vi "Abort Sequence-Ganging.vi"(8 "error in":errorcluster, 11 "Abort Sequence - Ganging":T1) -> (0 "error out":errorcluster)   [LabVIEW 2021]
doc: "Abort the sequence and if error resets the device for ganging configuration."
uses:
  controls/Abort Sequence-Ganging.ctl
  channel ganging/shared subVIs/ctl/NIDCPower_channel_ganging - ctl - ganged config.ctl
  channel ganging/shared subVIs/ctl/NIDCPower_channel_ganging - ctl - channel mode.ctl
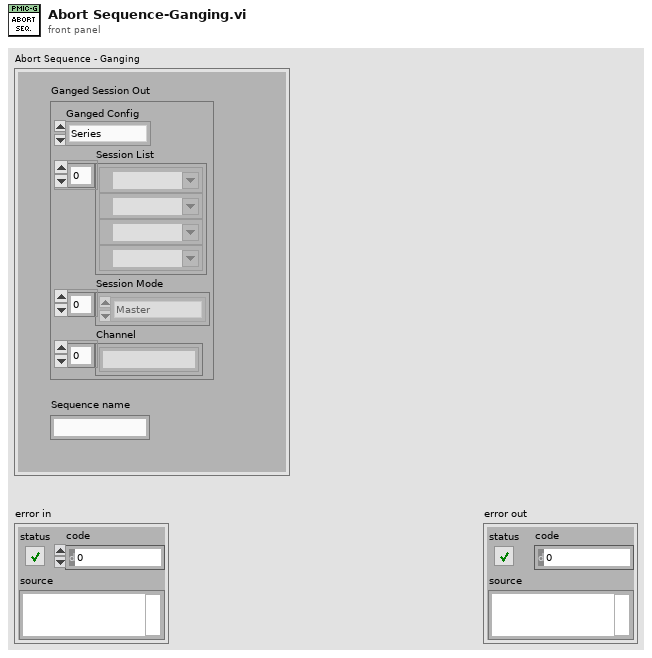
[diagram p1: front panel]
types:
  T1 = typedef "Abort Sequence-Ganging.ctl" = cluster{"Ganged Session Out":cluster{"Ganged Config":T2, "Session List":refnum<k15>[], "Session Mode":T3[], "Channel":string[]}, "Sequence name":string}
  T2 = typedef "NIDCPower_channel_ganging - ctl - ganged config.ctl" = enum32{"Series", "Parallel", "Manual"}
  T3 = typedef "NIDCPower_channel_ganging - ctl - channel mode.ctl" = enum32{"Master", "Slave", "Slave - Inverted"}
  T4 = cluster{"Ganged Config":T2, "Session List":refnum<k15>[], "Session Mode":T3[], "Channel":string[]}
  T5 = typedef "NIDCPower_channel_ganging - ctl - ganged session.ctl" = cluster{"Ganged Config":T2, "Session List":refnum<k15>[], "Session Mode":T3[], "Channel":string[]}
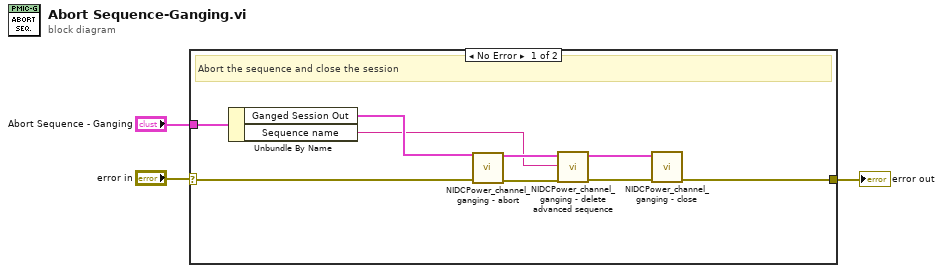
[diagram p0: block diagram]
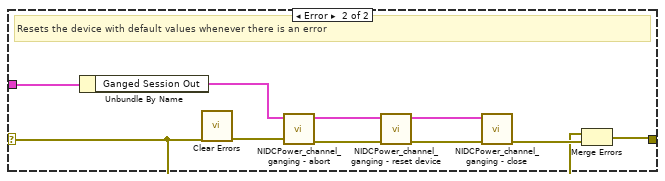
[diagram p2: hidden frame]
diagram:
  n1 = case shown="No Error" "error in" {
    selector: "error in" -> [w7 w14]
    tunnel: "Abort Sequence - Ganging" -> [w12 w22]
    tunnel: [w8 w13] -> w2
    frame No Error {
      # "Abort the sequence and close the session"
      n2 = Unbundle By Name(w12) -> ("Ganged Session Out"=w11:T4, "Sequence name"=w4:string)
      n3 = call "NIDCPower_channel_ganging - abort.vi"("error in (no error)"=w7, "Ganged Session In"=w11) -> ("error out"=w6:errorcluster, "Ganged Session Out"=w10:T5)  [unwired: 8 in]
      n4 = call "NIDCPower_channel_ganging - delete advanced sequence.vi"("error in (no error)"=w6, "sequence name"=w4, "Ganged Session In"=w10) -> ("error out"=w5:errorcluster, "Ganged Session Out"=w9:T5)  [unwired: 7 in]
      n5 = call "NIDCPower_channel_ganging - close.vi"("error in (no error)"=w5, "Ganged Session In"=w9) -> ("error out"=w8:errorcluster)  [unwired: 9 in]
    }
    frame Error {
      # "Resets the device with default values whenever there is an error"
      n6 = Unbundle By Name(w22) -> ("Ganged Session Out"=w17:T4)
      n7 = call <vilib>:"Clear Errors.vi"("error in (no error)"=w14) -> ("error out"=w16:errorcluster)  [unwired: 5 in, 1 out]
      n8 = call "NIDCPower_channel_ganging - abort.vi"("error in (no error)"=w16, "Ganged Session In"=w17) -> ("error out"=w20:errorcluster, "Ganged Session Out"=w21:T5)  [unwired: 8 in]
      n9 = call "NIDCPower_channel_ganging - reset device.vi"("error in (no error)"=w20, "Ganged Session In"=w21) -> ("error out"=w18:errorcluster, "Ganged Session Out"=w19:T5)  [unwired: 8 in]
      n10 = call "NIDCPower_channel_ganging - close.vi"("error in (no error)"=w18, "Ganged Session In"=w19) -> ("error out"=w15:errorcluster)  [unwired: 9 in]
      n11 = Merge Errors(w14, w15) -> (w13:errorcluster)
    }
  }
  "error out" <- w2
